vi "DRAM FPGA.vi"() -> ()   [LabVIEW 2014]
doc: "This FPGA VI illustrates use of the FFT Express VI in the <b>Single Channel, Multiple Samples</b> mode.\n\nThe entire data pipeline uses a handshaking protocol to ensure that no data is lost, by throttling upstream nodes if any node is not ready to receive data. If the pipeline is too slow (as determined by the host VI DMA Read loop), the Sine Wave FIFO will eventually overflow, returning <b>Timed Out?</b> and notifying the host UI."
uses:
  <instrlib>/_niInstr/Streaming/v1/Common/Stream State.ctl
  <vilib>/Platform/TimedLoop/XDataNode/timing_clust.ctl
  <vilib>/Platform/TimedLoop/XDataNode/nitl_modes.ctl
  <vilib>/Platform/TimedLoop/XDataNode/wakeup.ctl
  <vilib>/rvi/Emulation/niFpgaSctlEmulationGetInTimedLoop.vi
  <vilib>/rvi/Emulation/niFpgaEmulationReportErrorSimple.vi
  <vilib>/rvi/Emulation/niFpgaGetClockAttributes.vi
  <vilib>/rvi/Emulation/niFpgaCriticalErrorInLSC.vi
  <instrlib>/_niInstr/Data Formatting/v1/FPGA/Private/Convert/Boolean Array to U64 Array.vi
  <vilib>/rvi/interface/RandomDataEmulation/niFpgaRandomDataHandleErrors.vi
  <instrlib>/_niInstr/Data Formatting/v1/FPGA/Private/Convert/U16 array to Boolean Array.vi
  <vilib>/Platform/TimedLoop/XDataNode/XDataNode.xnode
  <vilib>/rvi/DataTransferAndStorage/Container/XNode/niFpgaContainer.xnode
  <vilib>/rvi/interface/RandomDataEmulation/nirviRandomDataFpgaReadWriteTemplate.vi
  <vilib>/Platform/TimedLoop/XDataNode/XDNodeRunTimeDep.lvlib
  <instrlib>/_niInstr/Streaming/v1/FPGA/niInstr Streaming v1 FPGA.lvlib
  <instrlib>/_niInstr/Data Formatting/v1/FPGA/niInstr Data Formatting v1 FPGA.lvlib
  K7 DRAM FIFO.lvclass
  <instrlib>/_niInstr/Streaming/v1/Common/niInstr Streaming v1 Common.lvlib
panel:
  in  "read grant time (clocks)":u16=100
  in  "write grant time (clocks)":u16=100
  in  "Tab Control":enum32{"Stream 0", "Stream 1"}(tab)
  in  "stream.num samples 0":u64
  out "stream.state 0":T1
  out "stream.samples transferred 0":u64
  in  "stream.request state 0":T1
  out "stream.metadata 0":u64
  out "stream.metadata 1":u64
  in  "stream.request state 1":T1
  out "stream.samples transferred 1":u64
  out "stream.state 1":T1
  in  "stream.num samples 1":u64
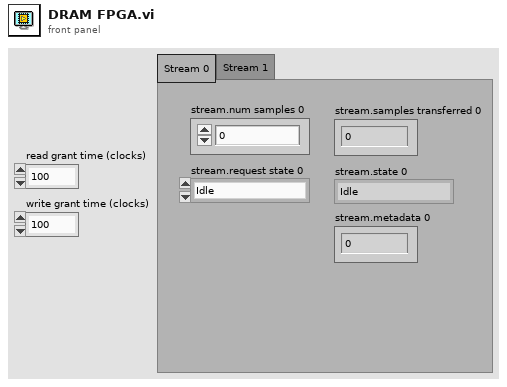
[diagram p1: front panel]
types:
  T1 = typedef "niInstr Streaming v1 Common.lvlib/Stream State.ctl" = enum8{"Idle", "Finite Transfer", "Continuous", "Done", "Error", "Not Ready", "Cancel"}
  T2 = typedef "XDNodeRunTimeDep.lvlib/timing_clust.ctl" = cluster{"Expected End [f-1]":u64, "Actual End [f-1]":u64, "Finished Late? [f-1]":bool, "Expected End [i-1]":u64, "Actual End [i-1]":u64, "Finished Late? [i-1]":bool, "Expected Start [i]":u64, "Actual Start [i]":u64, "Expected Start [f]":u64, "Actual Start [f]":u64, "Source Name":string, "Structure Name":string, "Period":i64, "Deadline":i64, "Offset":i64, "Start":i64, "Priority":i32, "Timeout":i32, "Mode":T3, "Wakeup Reason":T4, "Error":errorcluster, "Source Type":string, "Secondary Source Type":string, "Global End Time":u64, "Global Start Time":u64, "Frame Duration":u64, "Iteration Duration":u64, "Assigned CPU":i32, "I/O Scan Engine Mode":u32}
  T3 = typedef "XDNodeRunTimeDep.lvlib/nitl_modes.ctl" = enum32{"No Change", "Process missed periods, maintain original phase", "Discard missed periods, maintain original phase", "Process missed periods, ignore original phase", "Discard missed periods, ignore original phase"}
  T4 = typedef "XDNodeRunTimeDep.lvlib/wakeup.ctl" = enum32{"Normal", "Aborted", "Asynchronous wakeup", "Timing source error", "Timed loop error", "Timeout"}
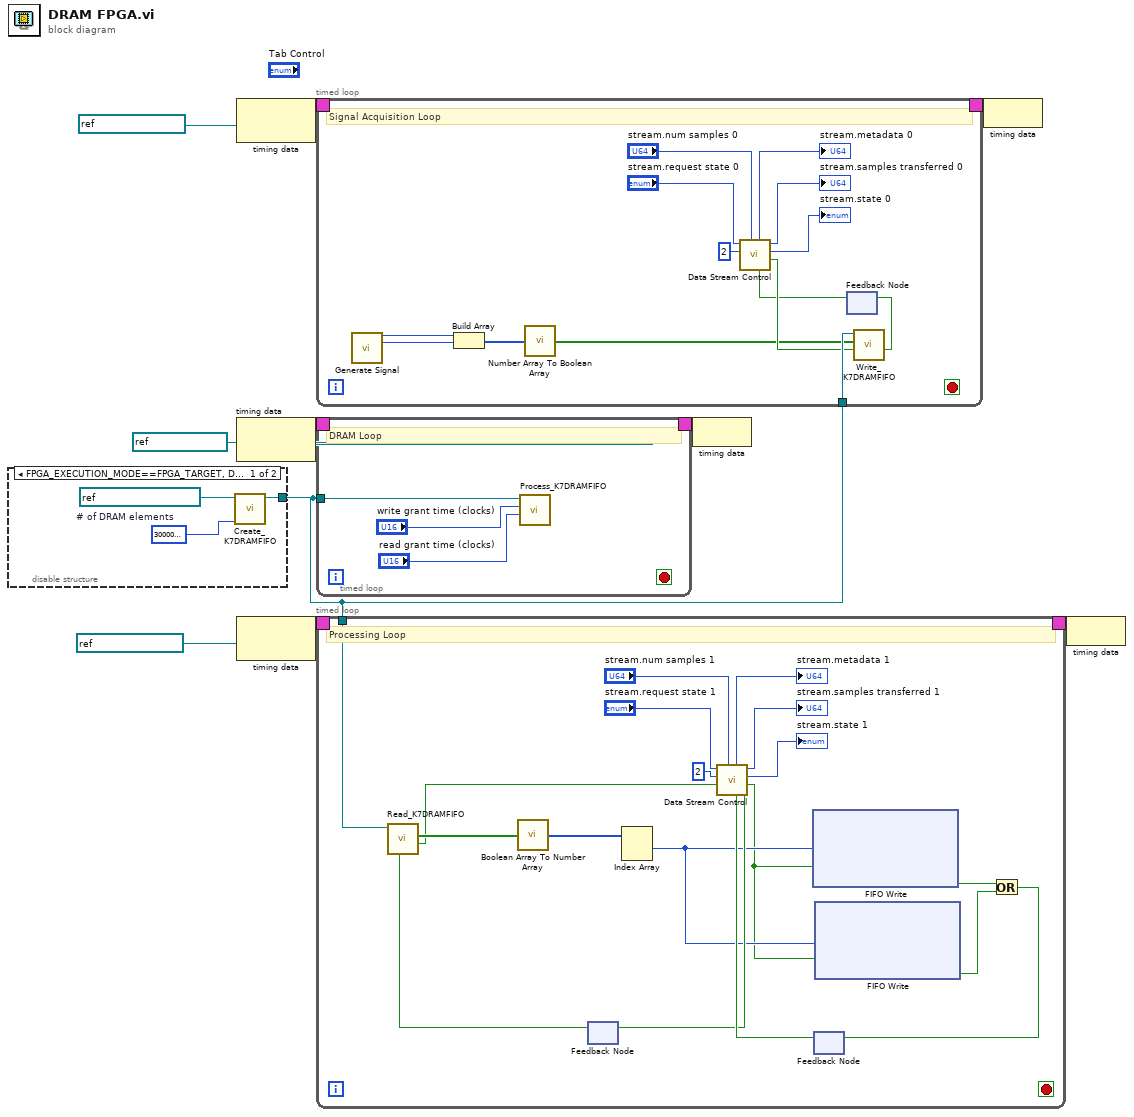
[diagram p0: block diagram]
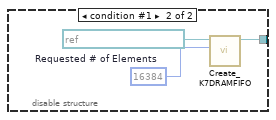
[diagram p2: hidden frame]
diagram:
  n1 = disable-structure shown="FPGA_EXECUTION_MODE==FPGA_TARGET, Default" {
    disable-tunnel: [w13 w14] -> w1
    frame condition #0 (active) {
      w11 = u32 300000000  # # of DRAM elements
      n2 = call "Create_K7DRAMFIFO.vi"("Requested # of Elements"=w11, "DRAM Bank 1 Ref"=refnum<k21> "DRAM FIFO 300M" ("memory in")) -> ("DRAM FIFO Ref Out"=w13:refnum<class "K7 DRAM FIFO.lvclass">)  [unwired: 9 in]
    }
    frame condition #1 {
      w15 = u32 16384  # Requested # of Elements
      n3 = call "Create_K7DRAMFIFO.vi"("DRAM Bank 2 Ref"=w15, "DRAM Bank 1 Ref"=refnum<k21> "DRAM FIFO 16384" ("memory in")) -> ("DRAM FIFO Ref Out"=w14:refnum<class "K7 DRAM FIFO.lvclass">)  [unwired: 9 in]
    }
  }
  n4 = node-c288(refnum<k21> "100 MHz Clock" ("Source Name")) -> (w8:T2)
  n5 = node-c288(refnum<k21> "DRAM Clock" ("Source Name")) -> (w5:T2)
  n6 = node-c288(refnum<k21> "200 MHz Clock" ("Source Name")) -> (w10:T2)
  n7 = timed-loop {
    timing: w8 -> [_]
    timing-out: [_] -> w7
    tunnel: w1 -> [w21]
    stop <- _ stop-if-true
    # "Signal Acquisition Loop"
    n8 = call "Generate Signal.vi"() -> ("AI N-1"=w23:i16, "AI N"=w22:i16)  [unwired: 14 in]
    n9 = Build Array(w23, w22) -> (w24:i16[])
    n10 = call-poly <instrlib>:"Number Array To Boolean Array.vi"("data in"=w24) -> ("data out"=w17:bool[])  [unwired: 14 in]
    n11 = feedback #1() -> (w18:bool)  [unwired: 1 in]
    n12 = call <instrlib>:"Data Stream Control.vi"("ready for input?"=w18, "stream.num samples 0"="stream.num samples 0", "element count"=u16 2, "stream.request state 0"="stream.request state 0") -> ("send data"=w20:bool, "stream.state 0"=→"stream.state 0":T1, "stream.samples transferred 0"=→"stream.samples transferred 0":u64, "stream.metadata 0"=→"stream.metadata 0":u64)  [unwired: 3 in, 1 out]
    n13 = call "Write_K7DRAMFIFO.vi"("Input Valid"=w20, "Element"=w17, "DRAM FIFO Ref In"=w21) -> ("Ready for Input"=w19:bool)  [unwired: 7 in, 1 out]
    n14 = feedback-in #1(w19) -> ()
  }
  n15 = timed-loop {
    timing: w5 -> [_]
    timing-out: [_] -> w4
    tunnel: w1 -> [w33]
    stop <- _ stop-if-true
    # "DRAM Loop"
    n16 = call "Process_K7DRAMFIFO.vi"("read grant time (clock ticks)"="read grant time (clocks)", "write grant time (clock ticks)"="write grant time (clocks)", "DRAM FIFO Ref In"=w33) -> ()  [unwired: 9 in]
  }
  n17 = timed-loop {
    timing: w10 -> [_]
    timing-out: [_] -> w9
    tunnel: w1 -> [w48]
    stop <- _ stop-if-true
    # "Processing Loop"
    n18 = feedback #2() -> (w43:bool)  [unwired: 1 in]
    n19 = call "Read_K7DRAMFIFO.vi"("Ready for Output"=w43, "DRAM FIFO Ref In"=w48) -> ("Output Valid"=w45:bool, "Element"=w46:bool[])  [unwired: 7 in, 1 out]
    n20 = call-poly <instrlib>:"Boolean Array To Number Array.vi"("data in"=w46) -> ("data out"=w47:u64[])  [unwired: 14 in]
    n21 = Index Array(array=w47) -> (element #1=w42:u64)  [unwired: 2 in, 1 out]
    n22 = feedback #3() -> (w49:bool)  [unwired: 1 in]
    n23 = call <instrlib>:"Data Stream Control.vi"("ready for input?"=w49, "stream.num samples 0"="stream.num samples 1", "data valid"=w45, "element count"=u16 2, "stream.request state 0"="stream.request state 1") -> ("request data"=w44:bool, "send data"=w38:bool, "stream.state 0"=→"stream.state 1":T1, "stream.samples transferred 0"=→"stream.samples transferred 1":u64, "stream.metadata 0"=→"stream.metadata 1":u64)  [unwired: 2 in]
    n24 = feedback-in #2(w44) -> ()
    n25 = xnode ("FIFO Write")("Element"=w42, "Input Valid"=w38) -> ("Ready for Input"=w41:bool)  [unwired: 1 in, 1 out]
    n26 = xnode ("FIFO Write")("Element"=w42, "Input Valid"=w38) -> ("Ready for Input"=w40:bool)  [unwired: 1 in, 1 out]
    n27 = Or(x=w41, y=w40) -> (x .or. y?=w39:bool)
    n28 = feedback-in #3(w39) -> ()
  }
  n29 = node-c288(w4) -> ()
  n30 = node-c288(w7) -> ()
  n31 = node-c288(w9) -> ()
